vi "Present Data.vi"(8 "error in (no error)":errorcluster, 11 "List Seen Processes View Model In":refnum<class "Process Tree View Model.lvclass">) -> (0 "error out":errorcluster, 3 "List Seen Processes View Model Out":refnum<class "Process Tree View Model.lvclass">)   [LabVIEW 2020, in "Process Tree View Model.lvclass"]
uses:
  Process Tree View Model.lvclass
  Process Tree View Model.lvclass/Process Tree View Model.ctl
  Tree Helpers/Tag Tree/Tag Tree.lvclass
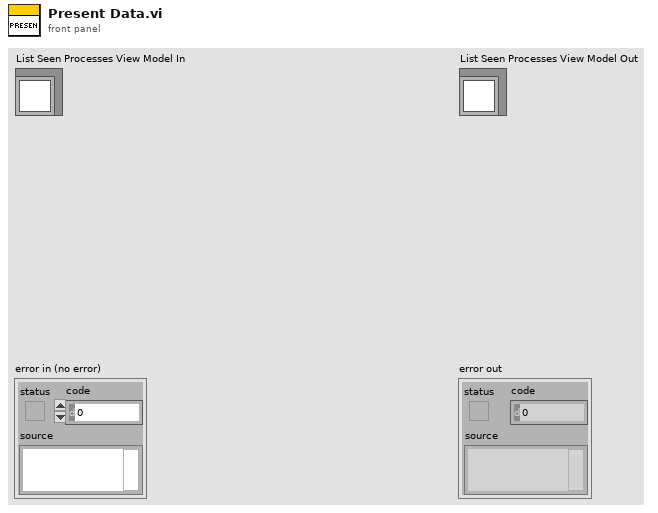
[diagram p1: front panel]
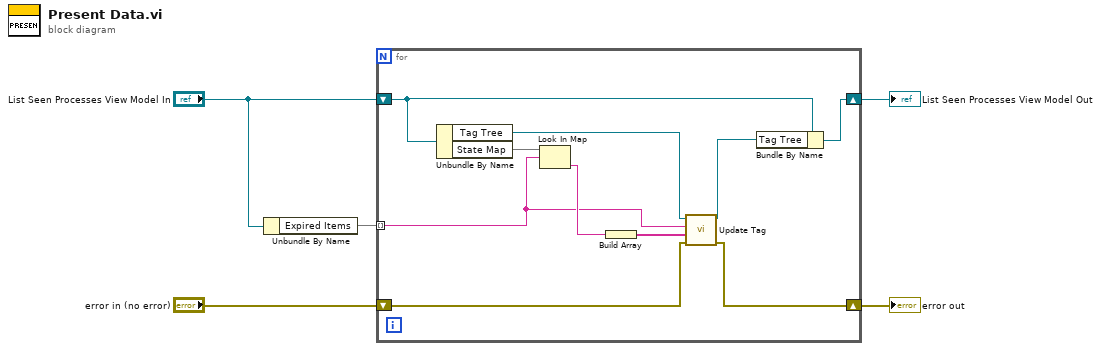
[diagram p0: block diagram]
diagram:
  n1 = Unbundle By Name("List Seen Processes View Model In") -> ("Expired Items"=w5:set{string})
  n2 = for {
    tunnel: w5 -> [w11] mode=indexing
    shift-right: [w7] -> w2
    shift-left: "error in (no error)" -> [w6]
    shift-right: [w9] -> w1
    shift-left: "List Seen Processes View Model In" -> [w10]
    n3 = Unbundle By Name(w10) -> ("Tag Tree"=w15:refnum<class "Tag Tree.lvclass">, "State Map"=w14:map{string, string})
    n4 = Look In Map(map=w14, key=w11) -> (value=w13:string)  [unwired: 1 in, 1 out]
    n5 = Build Array(w13) -> (w12:string[])
    n6 = call "Update Tag.vi"("error in (no error)"=w6, "Child Text"=w12, "Tag"=w11, "Tag Tree In"=w15) -> ("error out"=w7:errorcluster, "Tag Tree Out"=w8:refnum<class "Tag Tree.lvclass">)  [unwired: 6 in]
    n7 = Bundle By Name(cluster=w10, "Tag Tree"=w8) -> (w9:refnum<class "Process Tree View Model.lvclass">)
  }
  "error out" <- w2
  "List Seen Processes View Model Out" <- w1
